vi "serial.vi"() -> ()   [LabVIEW 2015]
doc: "This example performs writes and reads on a serial port, as directed by the user. You can press the Write and Read buttons, and change the Read Count, while the example is running.\n\nThe parameters set for the serial port must match the parameters of the connected instrument or device. In this example, the Read Count parameter specifies the number of bytes that the serial port reads. If there were more bytes at the port than the specified number, those bytes would not be read. If there were less bytes at the port than the specified number, you would receive a timeout error.\n\nThis example expands upon the flow control options for XON and XOFF, allowing the user to choose those control characters. Also, the user can enable or disable a termination character. Some devices require a termination character in order to identify the end of command strings. Some devices send a termination character to signify the end of data to be read. This example shows how you can end the Read operation once a termination character is detected in the buffer and/or append a termination character at the end of the Write data."
uses:
  <vilib>/Analysis/baseanly.llb/Mean (DBL).vi
  <vilib>/Instr/_visa.llb/VISA Configure Serial Port (Instr).vi
  <vilib>/express/express shared/transition.llb/Dynamic To Waveform Array.vi
  <vilib>/express/express arith-compare/Formula/Block/exnFormulaBlock how many pts in the wave.vi
  <vilib>/express/express shared/ex_Modify Signal Name.vi
  <vilib>/express/express shared/transition.llb/Waveform Array To Dynamic.vi
  <vilib>/express/express analysis/Spectral/Block/exnSpectralBlock spectral measurements peak poly.vi
  <vilib>/express/express analysis/Spectral/Block/exnSpectralBlock spectral measurements peak WFM.vi
  <vilib>/express/express arith-compare/Formula/XNode/ExpressFormulaBlockNode.xnode
  <vilib>/express/express analysis/Spectral/XNode/ExpressSpectralMeasurementsBlockNode.xnode
  <vilib>/ptbypt/NI_PtbyPt.lvlib
  <vilib>/Analysis/NI_AALBase.lvlib
panel:
  out "residual":dynamicdata(graph)
  out "Frequency":dbl
  out "R value":dbl
  out "SpO2 [%]":dbl
  out "RED LED":i32(graph)
  in  "Baud Rate":u32=115200
  out "IR DC (V)":dbl format="%0.2f"
  out "IR AC (Vrms)":dbl format="%0.2f"
  out "RED DC (V)":dbl format="%0.2f"
  out "RED AC (Vrms)":dbl format="%0.2f"
  out "AC/DC ir":dbl
  out "AC/DC red":dbl
  out "HR [bpm]":dbl
  out "Waveform Graph":dynamicdata(graph)
  out "IR LED":i32(graph)
  in  "Stop":bool
  in  "Read Count":u32=1000
  in  "VISA resource name":refnum<visa-resource-name>="COM5"
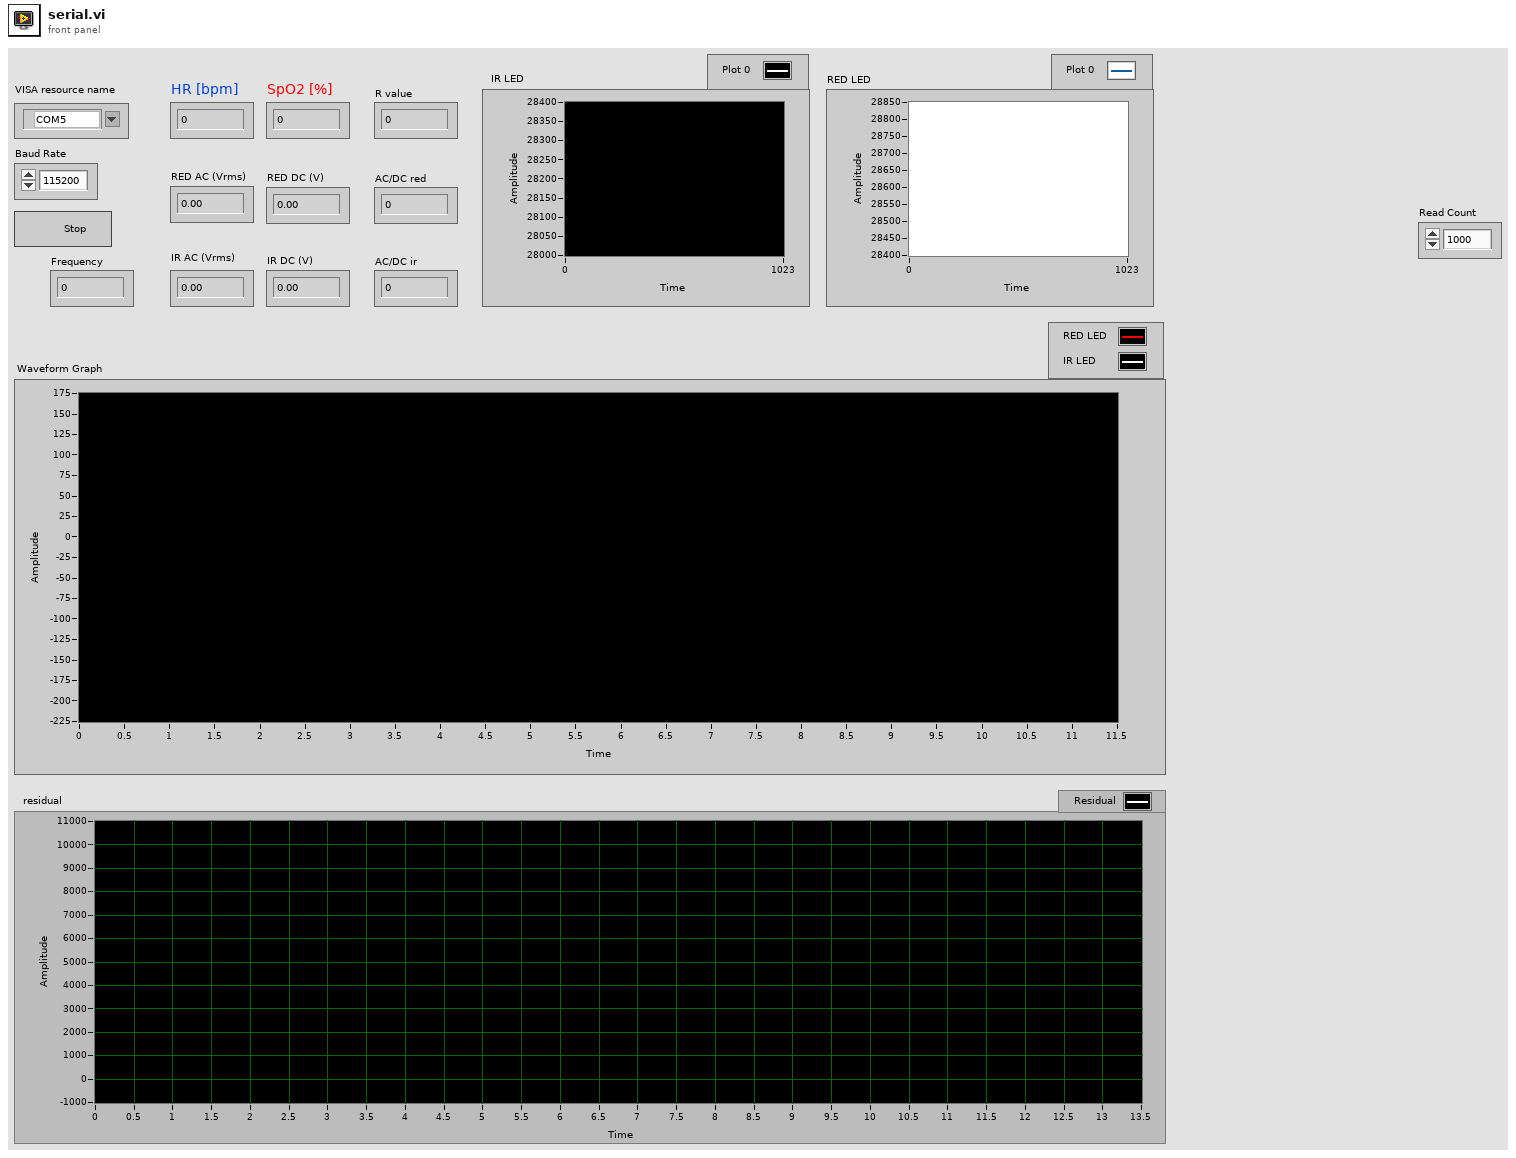
[diagram p1: front panel]
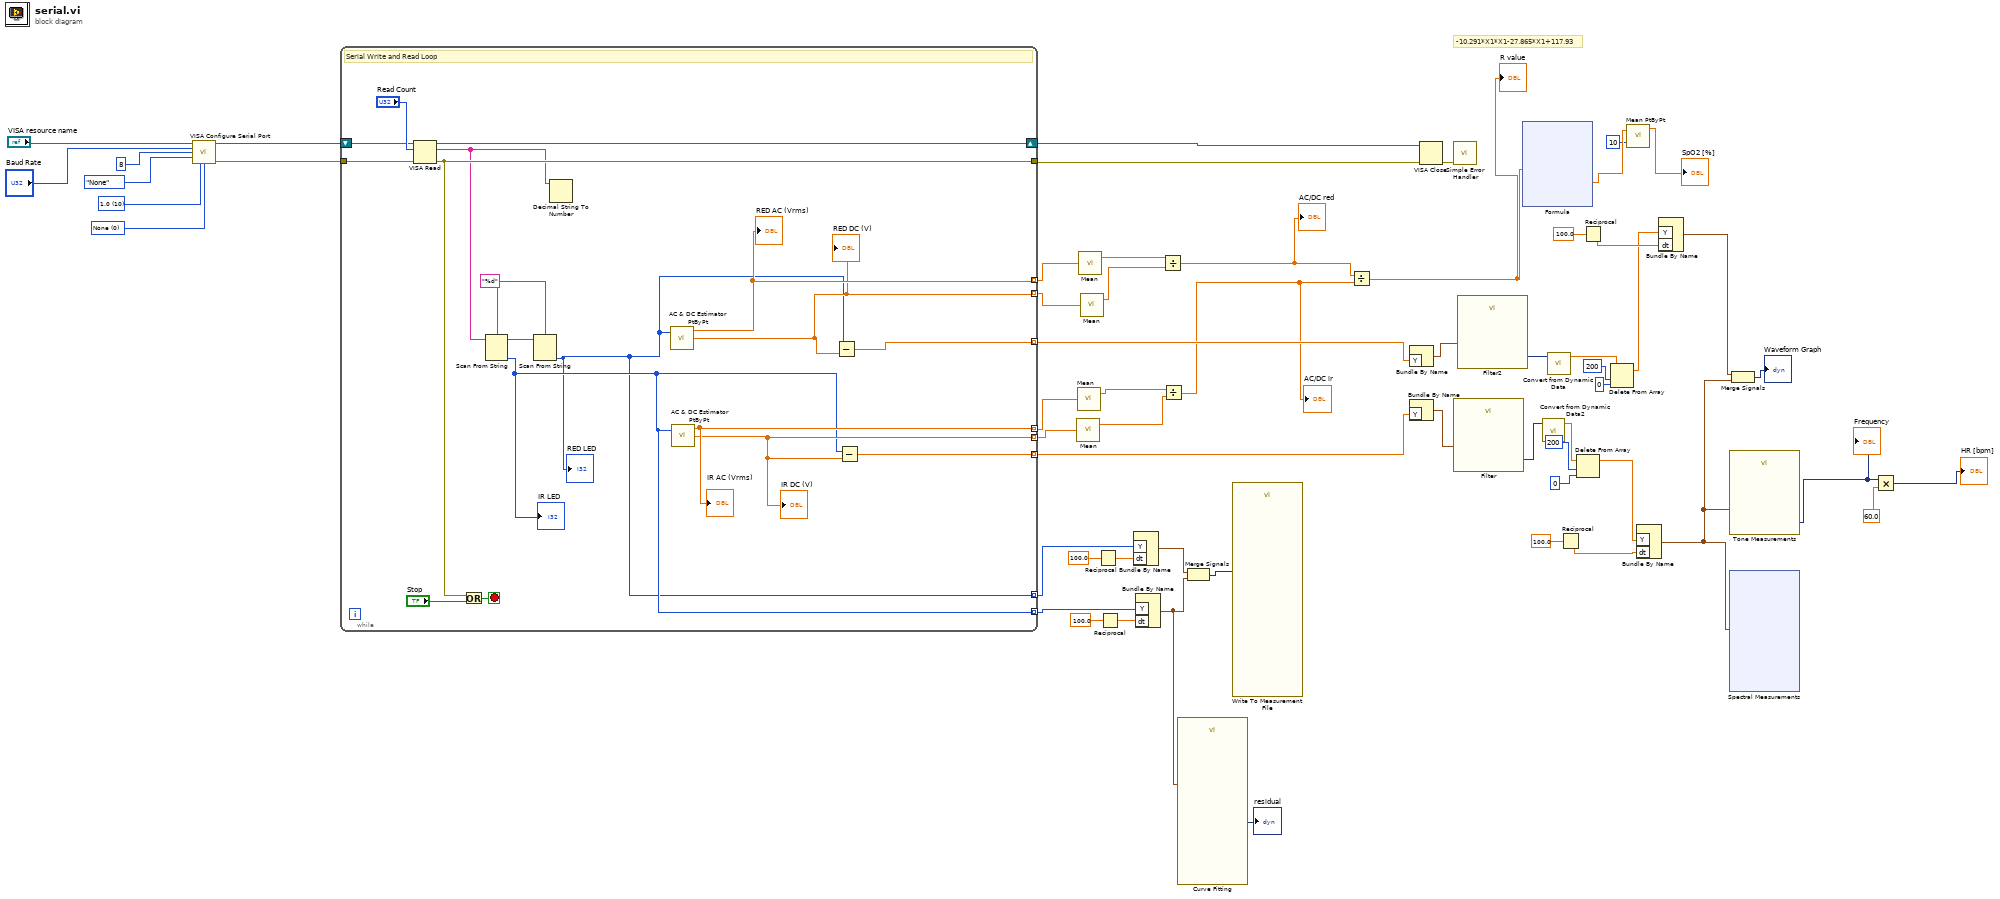
[diagram p0: block diagram]
diagram:
  w39 = u16 0 items=["None", "XON/XOFF", "RTS/CTS", "XON/XOFF & RTS/CTS", "DTR/DSR", "XON/XOFF & DTR/DSR"] ("flow control (0:none)")
  w40 = u16 10 items=["1.0"=10, "1.5"=15, "2.0"=20] ("stop bits (10: 1 bit)")
  # "-10.291*X1*X1-27.865*X1+117.93"
  n1 = call-poly "VISA Configure Serial Port"("VISA resource name"="VISA resource name", "baud rate (9600)"="Baud Rate", "data bits (8)"=u16 8, "parity (0:none)"=enum16{"None", "Odd", "Even", "Mark", "Space"}."None", "stop bits (10: 1 bit)"=w40, "flow control (0:none)"=w39) -> ("VISA resource name out"=w44:refnum<visa-resource-name>, "error out"=w43:errorcluster)  [unwired: 4 in, 4 out]
  n2 = while {
    shift-right: [w77] -> w56
    shift-left: w44 -> [w72]
    tunnel: w43 -> [w71]
    tunnel: [w75] -> w57
    tunnel: [w66] -> w50 mode=indexing
    tunnel: [w67] -> w51 mode=indexing
    tunnel: [w65] -> w24 mode=indexing
    tunnel: [w64] -> w22 mode=indexing
    tunnel: [w63] -> w20 mode=indexing
    tunnel: [w62] -> w19 mode=indexing
    tunnel: [w61] -> w8 mode=indexing
    tunnel: [w60] -> w12 mode=indexing
    stop <- w76 stop-if-true
    w68 = "%d" ("format string")
    # "Serial Write and Read Loop"
    n3 = VISA Read(VISA resource name=w72, byte count="Read Count", error in (no error)=w71) -> (VISA resource name out=w77:refnum<visa-resource-name>, read buffer=w70:string, error out=w75:errorcluster)  [unwired: 1 out]
    n4 = Or(x=w75, y="Stop") -> (x .or. y?=w76:bool)
    n5 = Scan From String(format string=w68, input string=w70) -> (remaining string=w69:string, output 1=w61:i32)  [unwired: 3 in, 2 out]
    "IR LED" <- w61
    n6 = Scan From String(format string=w68, input string=w69) -> (output 1=w60:i32)  [unwired: 3 in, 3 out]
    "RED LED" <- w60
    n7 = Decimal String To Number(string=w70) -> ()  [unwired: 2 in, 2 out]
    n8 = call <vilib>:"AC & DC Estimator PtByPt.vi"("signal"=w60) -> ("AC estimate (Vrms)"=w65:dbl, "DC estimate (V)"=w64:dbl)  [unwired: 2 in, 1 out]
    "RED AC (Vrms)" <- w65
    "RED DC (V)" <- w64
    n9 = call <vilib>:"AC & DC Estimator PtByPt.vi"("signal"=w61) -> ("AC estimate (Vrms)"=w63:dbl, "DC estimate (V)"=w62:dbl)  [unwired: 2 in, 1 out]
    "IR AC (Vrms)" <- w63
    "IR DC (V)" <- w62
    n10 = Subtract(x=w60, y=w64) -> (x-y=w67:dbl)
    n11 = Subtract(x=w61, y=w62) -> (x-y=w66:dbl)
  }
  n12 = call-poly <vilib>:"Mean.vi"("X"=w19) -> ("mean"=w17:dbl)  [unwired: 1 out]
  n13 = call-poly <vilib>:"Mean.vi"("X"=w20) -> ("mean"=w18:dbl)  [unwired: 1 out]
  n14 = call-poly <vilib>:"Mean.vi"("X"=w24) -> ("mean"=w23:dbl)  [unwired: 1 out]
  n15 = call-poly <vilib>:"Mean.vi"("X"=w22) -> ("mean"=w21:dbl)  [unwired: 1 out]
  n16 = Reciprocal(x=100.0) -> (1/x=w13:dbl)
  n17 = Reciprocal(x=100.0) -> (1/x=w10:dbl)
  n18 = Bundle By Name("Y"=w12, "dt"=w13) -> (w11:waveform(i32))  [unwired: 1 in]
  n19 = Bundle By Name("Y"=w8, "dt"=w10) -> (w2:waveform(i32))  [unwired: 1 in]
  n20 = Divide(x=w23, y=w21) -> (x/y=w26:dbl)
  "AC/DC red" <- w26
  n21 = Divide(x=w18, y=w17) -> (x/y=w25:dbl)
  "AC/DC ir" <- w25
  n22 = call "Curve Fitting"("Signals"=w2) -> ("residual"=→"residual":dynamicdata)  [unwired: 4 in, 6 out]
  n23 = Merge Signals(w11, w2) -> (w15:dynamicdata)
  n24 = call "Write To Measurement File"("Signals"=w15) -> ()  [unwired: 16 in, 3 out]
  n25 = Divide(x=w26, y=w25) -> (x/y=w27:dbl)
  "R value" <- w27
  n26 = Bundle By Name("Y"=w51) -> (w54:waveform(dbl))  [unwired: 1 in]
  n27 = Bundle By Name("Y"=w50) -> (w55:waveform(dbl))  [unwired: 1 in]
  n28 = VISA Close(VISA resource name=w56, error in (no error)=w57) -> (error out=w58:errorcluster)
  n29 = call <vilib>:"Simple Error Handler.vi"("error in (no error)"=w58) -> ()  [unwired: 1 in, 8 out]
  n30 = call "Filter"("Signal"=w55) -> ("Filtered Signal"=w7:dynamicdata)  [unwired: 9 in, 1 out]
  n31 = call "Filter2"("Signal"=w54) -> ("Filtered Signal"=w49:dynamicdata)  [unwired: 9 in, 1 out]
  n32 = xnode "Formula"("X1"=w27) -> ("Result"=w30:dbl)  [unwired: 1 in, 1 out]
  n33 = call "Convert from Dynamic Data2"("Dynamic Data Type"=w7) -> ("Array"=w47:dbl[])  [unwired: 3 in]
  n34 = call "Convert from Dynamic Data"("Dynamic Data Type"=w49) -> ("Array"=w48:dbl[])  [unwired: 3 in]
  n35 = Reciprocal(x=100.0) -> (1/x=w36:dbl)
  n36 = Delete From Array(array=w47, length=200, index=0) -> (array with subset deleted=w35:dbl[])  [unwired: 1 out]
  n37 = Reciprocal(x=100.0) -> (1/x=w33:dbl)
  n38 = Delete From Array(array=w48, length=200, index=0) -> (array with subset deleted=w32:dbl[])  [unwired: 1 out]
  n39 = call <vilib>:"Mean PtByPt.vi"("x"=w30, "sample length"=10) -> ("mean"=→"SpO2 [%]":dbl)  [unwired: 2 in, 1 out]
  n40 = Bundle By Name("Y"=w35, "dt"=w36) -> (w3:waveform(dbl))  [unwired: 1 in]
  n41 = Bundle By Name("Y"=w32, "dt"=w33) -> (w31:waveform(dbl))  [unwired: 1 in]
  n42 = call "Tone Measurements"("Signals"=w3) -> ("Frequency"=w4:dynamicdata)  [unwired: 9 in, 1 out]
  "Frequency" <- w4
  n43 = xnode "Spectral Measurements"("Signals"=w3) -> ()  [unwired: 1 in, 3 out]
  n44 = Merge Signals(w31, w3) -> (→"Waveform Graph":dynamicdata)
  n45 = Multiply(x=w4, y=60.0) -> (x*y=→"HR [bpm]":dynamicdata)
